vi "Cooling Tower Monitor v1_0.vi"() -> ()   [LabVIEW 2012]
panel:
  in  "Mixer":bool
  in  "stop":bool
  out "Resevoir Temp":dbl format="%.1g"
  out "Inlet Dry Bulb Temp":dbl format="%.1g"
  out "Inlet Wet Bulb Temp":dbl format="%.1g"
  out "Outlet Wet Bulb Temp":dbl format="%.1g"
  out "Outlet Dry Bulb Temp":dbl format="%.1g"
  out "Inlet Water Temp":dbl format="%.1g"
  out "Outlet Water Temp":dbl format="%.1g"
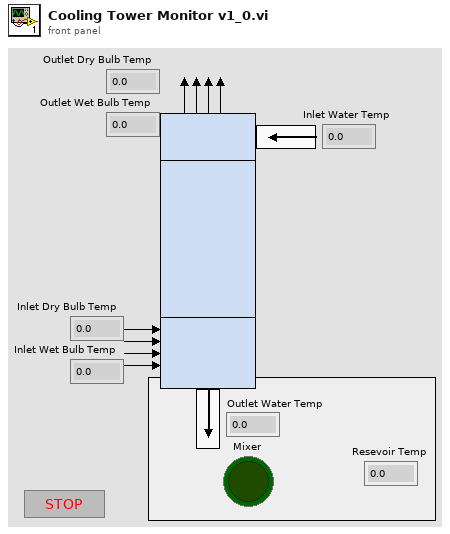
[diagram p1: front panel]
types:
  T1 = cluster{"Outlet Water Temp":dbl, "Inlet Water Temp":dbl, "Outlet Dry Bulb Temp":dbl, "Outlet Wet Bulb Temp":dbl, "Inlet Wet Bulb Temp":dbl, "Inlet Dry Bulb Temp ":dbl, "Resevoir Temp":dbl}
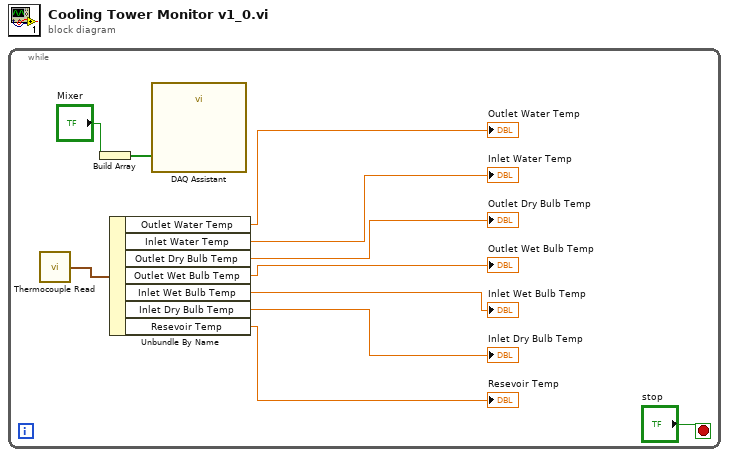
[diagram p0: block diagram]
diagram:
  n1 = while {
    stop <- "stop" stop-if-true
    n2 = call "Thermocouple Read.vi"() -> ("Cluster"=w11:T1)  [unwired: 1 in]
    n3 = Build Array("Mixer") -> (w1:bool[])
    n4 = Unbundle By Name(w11) -> ("Outlet Water Temp"=→"Outlet Water Temp":dbl, "Inlet Water Temp"=→"Inlet Water Temp":dbl, "Outlet Dry Bulb Temp"=→"Outlet Dry Bulb Temp":dbl, "Outlet Wet Bulb Temp"=→"Outlet Wet Bulb Temp":dbl, "Inlet Wet Bulb Temp"=→"Inlet Wet Bulb Temp":dbl, "Inlet Dry Bulb Temp"=→"Inlet Dry Bulb Temp":dbl, "Resevoir Temp"=→"Resevoir Temp":dbl)
    n5 = call "DAQ Assistant"("data"=w1) -> ()  [unwired: 17 in, 2 out]
  }
